vi "PWM.Measure.Digital.Convert.vi"(11 "Result":T2) -> (3 "Analyzed":T1)   [LabVIEW 2015, in "Speciality FPGA IO.lvlib"]
uses:
  Speciality FPGA IO.lvlib
  Types/PWM.Measure.Digital.Result.ctl
  Types/PWM.Measure.Digital.Analyzed.ctl
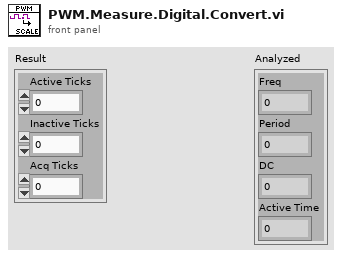
[diagram p1: front panel]
types:
  T1 = typedef "Speciality FPGA IO.lvlib/PWM.Measure.Digital.Analyzed.ctl" = cluster{"Freq":sgl, "Period":sgl, "DC":sgl, "Active Time":sgl}
  T2 = typedef "Speciality FPGA IO.lvlib/PWM.Measure.Digital.Result.ctl" = cluster{"Active Ticks":u32, "Inactive Ticks":u32, "Acq Ticks":u32}
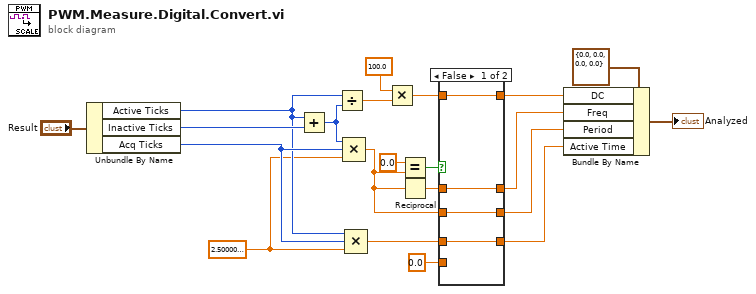
[diagram p0: block diagram]
diagram:
  w10 = sgl 2.5e-08 ("y")
  n1 = Unbundle By Name("Result") -> ("Active Ticks"=w17:u32, "Inactive Ticks"=w21:u32, "Acq Ticks"=w19:u32)
  n2 = Add(x=w17, y=w21) -> (x+y=w12:u32)
  n3 = Divide(x=w17, y=w12) -> (x/y=w13:sgl)
  n4 = Compound Arithmetic op=MULTIPLY(w12, w19, w10) -> (w14:sgl)
  n5 = Compound Arithmetic op=MULTIPLY(w17, w19, w10) -> (w11:sgl)
  n6 = Multiply(x=sgl 100.0, y=w13) -> (x*y=w2:sgl)
  n7 = Equal?(x=sgl 0.0, y=w14) -> (x = y?=w9:bool)
  n8 = Reciprocal(x=w14) -> (1/x=w15:sgl)
  n9 = case shown="False" w9 {
    tunnel: [w22 w26] -> w5
    tunnel: [w23 w26] -> w4
    tunnel: [w25 w26] -> w6
    tunnel: w14 -> [w25 _]
    tunnel: [w24 w26] -> w7
    tunnel: w11 -> [w24 _]
    tunnel: w2 -> [w23 _]
    tunnel: w15 -> [w22 _]
    tunnel: sgl 0.0 ("x") -> [_ w26]
    frame False {
    }
    frame True {
    }
  }
  n10 = Bundle By Name(cluster=T1 {"Freq"=0.0, "Period"=0.0, "DC"=0.0, "Active Time"=0.0} ("Analyzed"), "DC"=w4, "Freq"=w5, "Period"=w6, "Active Time"=w7) -> (→"Analyzed":T1)
